vi "Clear Limit.vi"(8 "error in (no error)":errorcluster, 10 "Limit (1: Limit 1)":i32(ring)=1 items=["Limit 1"=1, "Limit 2"=2], 11 "VISA resource name":refnum<visa-resource-name>) -> (0 "error out":errorcluster, 3 "VISA resource name out":refnum<visa-resource-name>)   [LabVIEW 2016, in "Keithley 2182.lvlib"]
doc: "Clears limit fail indication."
uses:
  Keithley 2182.lvlib
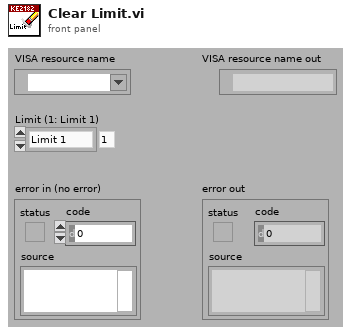
[diagram p1: front panel]
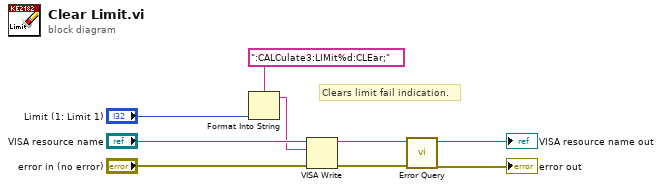
[diagram p0: block diagram]
diagram:
  # "Clears limit fail indication."
  n1 = Format Into String(format string=":CALCulate3:LIMit%d:CLEar;", "Limit (1: Limit 1)") -> (resulting string=w1:string)  [unwired: 2 in, 1 out]
  n2 = VISA Write(VISA resource name="VISA resource name", write buffer=w1, error in (no error)="error in (no error)") -> (VISA resource name out=w7:refnum<visa-resource-name>, error out=w6:errorcluster)  [unwired: 1 out]
  n3 = call "Error Query.vi"("error in (no error)"=w6, "VISA resource name"=w7) -> ("error out"=→"error out":errorcluster, "VISA resource name out"=→"VISA resource name out":refnum<visa-resource-name>)  [unwired: 6 in, 2 out]
